vi "VisBx Anzeige_Paccar.vi"() -> ()   [LabVIEW 2020, in "Anlagenuebersicht.lvlib"]
uses:
  Seiten/Anlagenuebersicht/VisBx Anzeige/Anlagenuebersicht.lvlib
  Visualisierungs Elemente/Zahlen-Ausgabefeld.ctl
  Seiten/Anlagenuebersicht/Aktionen Ausgabefaelder einfaerben.ctl
  <vilib>/Utility/miscctls.llb/LVPointTypeDef.ctl
  Seiten/Anlagengrenzwerte/FGV Anlagengrenzwerte Aktionen.ctl
  Seiten/FT-IR/FGV FT-IR Gasliste Aktionen.ctl
  PNS/Aktionen FGV Grenzwerte.ctl
  Seiten/System Einstellungen V2/Aktioen FGV System.ctl
  Seiten/Anlagenuebersicht/VisBx Anzeige/Aktion FGV Ventile manuell schalten Crio.ctl
  Seiten/FT-IR/FGV FT-IR Diagnose Aktionen.ctl
  Messdaten/Aktionen FGV Messdaten.ctl
  Amium PNS/Aktion FGV Amium Daten.ctl
  PNS/Aktionen FGV Istwerte.ctl
  Stoerungen/Stoerungen Messgeraet/Aktionen Kommunikation Stoerung.ctl
  Funktionstasten/FGV Erweiterte Bedienung Aktion.ctl
  PNS/Aktion FGV Ventile manuell steuern.ctl
  PNS/Aktionen FGV Loopkennung.ctl
  Funktionstasten/Funktionstasten-Aktion.ctl
  <vilib>/picture/picture.llb/Draw True-Color Pixmap.vi
  Seiten/Erweiterte Konfig/Konfig CG-Check/CG-Test.vi
  Seiten/Anlagenuebersicht/VisBx Anzeige/VisBx Anzeige.lvlib
  Seiten/Anlagenuebersicht/VisBx Anzeige/TDMS laden/TDMS laden.lvlib
  Allgemein/allgemeine Sub-VIs.lvlib
  cRIO/PC/Kommunikation mit cRIO.lvlib
  Seiten/FT-IR/FT-IR.lvlib
  Stoerungen/Stoerungen.lvlib
  Seiten/Anlagengrenzwerte/Anlagengrenzwerte.lvlib
  Funktionstasten/Funktionstasten.lvlib
  Messdaten/Messdaten.lvlib
  PNS/PNS.lvlib
  Seiten/System Einstellungen V2/System Einstellungen V2.lvlib
  Seiten/Erweiterte Konfig/Konfig CG-Check/CG-Check Konfig.lvlib
  Amium PNS/Amium PNS.lvlib
  Amium PNS/Anlagenuebersicht_amium2.vi
  Passwortverwaltung/Passwort.lvlib
  Passwortverwaltung/FGV Passwort Aktion.ctl
panel:
  in  "21Y6":bool
  in  "Eingang 4":bool
  in  "Eingang 3":bool
  in  "Manueller Betrieb":u16(ring) caption="Manual Mode" items=["Normal Mode", "TESTMODE!!!!"]
  in  "11Y2":bool
  in  "11Y3":bool
  in  "12Y1":bool
  in  "11Y7":bool
  in  "11Y6":bool
  in  "21Y5":bool
  in  "20Y1":bool
  in  "20Y5":bool
  in  "21Y1":bool
  in  "20Y8":bool
  in  "20Y7":bool
  in  "20Y6":bool
  in  "20Y4":bool
  in  "20Y3":bool
  in  "20Y2":bool
  in  "23Y4":bool
  in  "23Y3":bool
  in  "22Y2":bool
  in  "23Y6":bool
  in  "11Y5":bool
  in  "22Y1":bool
  out "16B1":string="LS\n\n-16B1" caption="-21Y8"
  out "N2Exh 2":string="N2\nEXH"
  out "-22Y3 50l 2":string="-22Y3" caption="-21Y8"
  out "17B3 50l":string="LS\n\n-17B3" caption="-21Y8"
  out "17B2 50l":string="LS\n\n-17B2" caption="-21Y8"
  out "16B2 50l":string="LS\n\n-16B2" caption="-21Y8"
  out "16B2":string="LS\n\n-16B2" caption="-21Y8"
  out "-22Y1 50l":string="-22Y1" caption="-21Y8"
  out "-22Y1":string="-22Y1" caption="-21Y8"
  out "PR0,2":string="PR\n0,3bar"
  out "PA3":string="PA\n3"
  out "N2Exh":string="N2\nEXH"
  out "-23Y8":string="-23Y8"
  out "-21Y7":string="-21Y7"
  out "-21Y8":string="-21Y8"
  out "Umgebungstemperatur:":T1 caption="Ambient temperature:" format="%.1f"
  out "Boolesch":bool
  out "HL Ext. SP1:":T1 format="%.1f"
  in  "VFS":bool
  in  "VFS - Inaktiv":bool caption="VFS - Inactive"
  in  "VFS - FEHLER":bool caption="VFS - ERROR"
  in  "VFS - Aktiv":bool=TRUE caption="VFS - Active"
  out "kPa":T1 caption="Messgasdruck Amium"
  out "Durchflussblock":T1 caption="Durchflussblock:" format="%.1f"
  out "Druck Filterblock:":T1
  in  "CG-Test":bool caption="Dichtheitstest"
  out "Umgebungsdruck:":T1 caption="Ambient pressure:"
  out "Druck Ausgang:":T1 caption="Pressure outlet:"
  out "Durchfluss Bypass:":T1 caption="Flow Bypass:" format="%.1f"
  out "HL zu FID:":T1 format="%.1f"
  out "Filterblock PNS":T1 caption="Filterblock:" format="%.1f"
  out "Heizleitung SP2:":T1 caption="HL SP2:" format="%.1f"
  out "Heizleitung SP1:":T1 caption="HL SP1:" format="%.1f"
  out "Gaskühler 2":T1 caption="Gascooler:" format="%.1f"
  out "Gaskühler":T1 caption="Gascooler:" format="%.1f"
  out "Flow PMA:":T1 format="%.1f"
  out "Taupunkt":T1 caption="Dewpoint:" format="%.1f"
  out "Druck Kalter Block":T1 caption="Pressure Cold Block:"
  out "O2":T1 caption="O2:" format="%.2f"
  out "H2O":T1 format="%.2f"
  out "HC":T1 caption="HC:"
  in  "N2 zu PNS":bool
  out "Heizung VFE2:":T1 format="%.1f"
  out "HL Ext. SP2:":T1 format="%.1f"
  out "Schaltschrank:":T1 caption="Cabinet temperature:" format="%.1f"
  out "Druck CalGas:":T1 caption="Pressure CalGas:" format="%.1f"
  out "HL zu Filter:":T1 caption="HL to Filter:" format="%.1f"
  out "HL zu FT-IR:":T1 caption="HL to FT-IR:" format="%.1f"
  out "Filter:":T1 format="%.1f"
  out "Pumpe:":T1 caption="Pump:" format="%.1f"
  out "Betriebsstunden Pumpe:":T1 caption="Operating hours (measure):" format="%.1f"
  out "Betriebsstunden Anlage:":T1 caption="Operating hours (unit / FT-IR):" format="%.1f"
  out "Temp. Messzelle:":T1 caption="Temp. Gascell:" format="%.1f"
  out "Eingangsdruck FT-IR:":T1 caption="Pressure FT-IR:" format="%.3f"
  out "Durchfluss FT-IR:":T1 caption="Flow FT-IR:" format="%.1f"
  out "Aktive Störungen":string[](array[string]) caption="Errors"
  in  "Fehler":string="Die Umgebungsvariable besitzt\nnicht den selben Datentyp wie\ndie TDMS-Datei."
  out "Bild":picture
  # "Process Chart"
  # "-23Y6"
  # "-35B5"
  # "-23Y3"
  # "SPAN 1"
  # "PS"
  # "-22Y2"
  # "0-10"
  # "-20Y2"
  # "bar"
  # "-23Y4"
  # "SPAN 2"
  # "N2.....Nitrogen gaseous\nCA.....Compressed air\nCG.....Cal. Gas\nAA.....Ambient air\nPA.....Purge air FT-IR\nZG.....ZeroGas\n\nPR....Pressure regulator\nPS....Pressure switch\nFS....Flow controller\nLS....Levelsensor\nFM...Flow Sensor"
  # "PR12"
  # "-17S5"
  # "-35B1"
  # "-20Y3"
  # "SPAN 3"
  # "FM"
  # "-43Y1"
  # "-20Y4"
  # "S"
  # "SPAN 4"
  # "-21Y5"
  # "FTIR"
  # "-20Y5"
  # "SPAN 5"
  # "-20Y6"
  # "SPAN 6"
  # "-20Y7"
  # "SPAN 7"
  # "Reservoir 5l"
  # "-20Y8"
  # "SPAN 8"
  # "-35B2"
  # "-21Y1"
  # "ZeroGas"
  # "-11Y7"
  # "-11Y3"
  # "SP1"
  # "-11Y5"
  # "-11Y6"
  # "SP2"
  # "-11Y2"
  # "-12Y1"
  # "Exhaust"
  # "7A1"
  # "P out"
  # "CA to PNS"
  # "-17B8"
  # "CA in"
  # "min 4bar"
  # "-20Y1"
  # "PR01"
  # "-17S1"
  # "Purge in"
  # "-21Y6"
  # "-20Y8"
  # "°C"
  # "°C"
  # "-44Y1"
  # "-21Y8"
  # "-23Y8"
  # "-21Y7"
  # "°C"
  # "mbar"
  # "-10M2"
  # "-20Y2"
  # "°C"
  # "-20Y4"
  # "-20Y6"
  # "-7M8"
  # "-35B10"
  # "-35B6"
  # "OP"
  # "1"
  # "PS"
  # "1bar"
  # "PR"
  # "2bar"
  # "CG"
  # "PNS"
  # "SPAN 1"
  # "-23Y1"
  # "SPAN 2"
  # "PS"
  # "-23Y2"
  # "SPAN 3"
  # "0-10"
  # "bar"
  # "-23Y3"
  # "-35B5"
  # "N2.....Nitrogen gaseous\nCA.....Compressed air\nCG.....Cal. Gas\nAA.....Ambient air\nPA.....Purge air FT-IR\n\nPR....Pressure regulator\nPS....Pressure switch\nFS....Flow controller\nLS....Levelsensor\nFM...Flow Sensor"
  # "-23Y4"
  # "-21Y5"
  # "-11Y7"
  # "-11Y3"
  # "SP1"
  # "-11Y5"
  # "-11Y6"
  # "SP2"
  # "-11Y2"
  # "-12Y1"
  # "-11Y8"
  # "EPR"
  # "5bar"
  # "CA"
  # "PNS"
  # "CG"
  # "PNS"
  # "N2"
  # "4-5"
  # "CG"
  # "PNS"
  # "N2"
  # "1"
  # "PR"
  # "2bar"
  # "PS"
  # "1bar"
  # "FS"
  # "3l"
  # "PR51"
  # "N2"
  # "1-2"
  # "LS"
  # "°C"
  # "CA"
  # "6"
  # "EPR"
  # "5bar"
  # "CA"
  # "PNS"
  # "ZG"
  # "2"
  # "CG"
  # "PNS"
  # "ZG"
  # "1"
  # "PR"
  # "2bar"
  # "PS"
  # "1bar"
  # "FS"
  # "3l"
  # "PR51"
  # "N2"
  # "1-2"
  # "OP"
  # "1"
  # "CA"
  # "1-2"
  # "CA"
  # "1"
  # "ZG"
  # "2"
  # "CA"
  # "2"
  # "ZG"
  # "1"
  # "FID"
  # "EXH"
  # "°C"
  # "°C"
  # "mbar"
  # "mbar"
  # "l/min"
  # "°C"
  # "FID"
  # "EXH"
  # "M2"
  # "PR02"
  # "PR"
  # "4bar"
  # "CA"
  # "FID"
  # "M6"
  # "PR06"
  # "M7"
  # "PR07"
  # "H2"
  # "FID"
  # "PR"
  # "1,2bar"
  # "SA"
  # "FID"
  # "PR"
  # "1,2bar"
  # "-27Y4"
  # "-27Y3"
  # "PR09"
  # "-35B8"
  # "CG"
  # "O2"
  # "PS"
  # "3,5bar"
  # "FR"
  # "1,5l"
  # "FID"
  # "FID"
  # "EXH"
  # "4 bar"
  # "CA"
  # "1,2bar"
  # "H2"
  # "1,2bar"
  # "SA"
  # "SPAN 2"
  # "SPAN 3"
  # "°C"
  # "°C"
  # "°C"
  # "°C"
  # "°C"
  # "l/min"
  # "°C"
  # "mbar"
  # "H"
  # "S"
  # "P"
  # "abs"
  # "PMD"
  # "%"
  # "-35B9"
  # "FM"
  # "S"
  # "-27Y2"
  # "CG O2"
  # "CG"
  # "O2"
  # "%"
  # "ppm"
  # "°C"
  # "°C"
  # "°C"
  # "bar"
  # "°C"
  # "°C"
  # "°C"
  # "°C"
  # "h"
  # "h"
  # "°C"
  # "atm"
  # "l/min"
  # "PR"
  # "5bar"
  # "PS"
  # "4bar"
  # "P"
  # "abs"
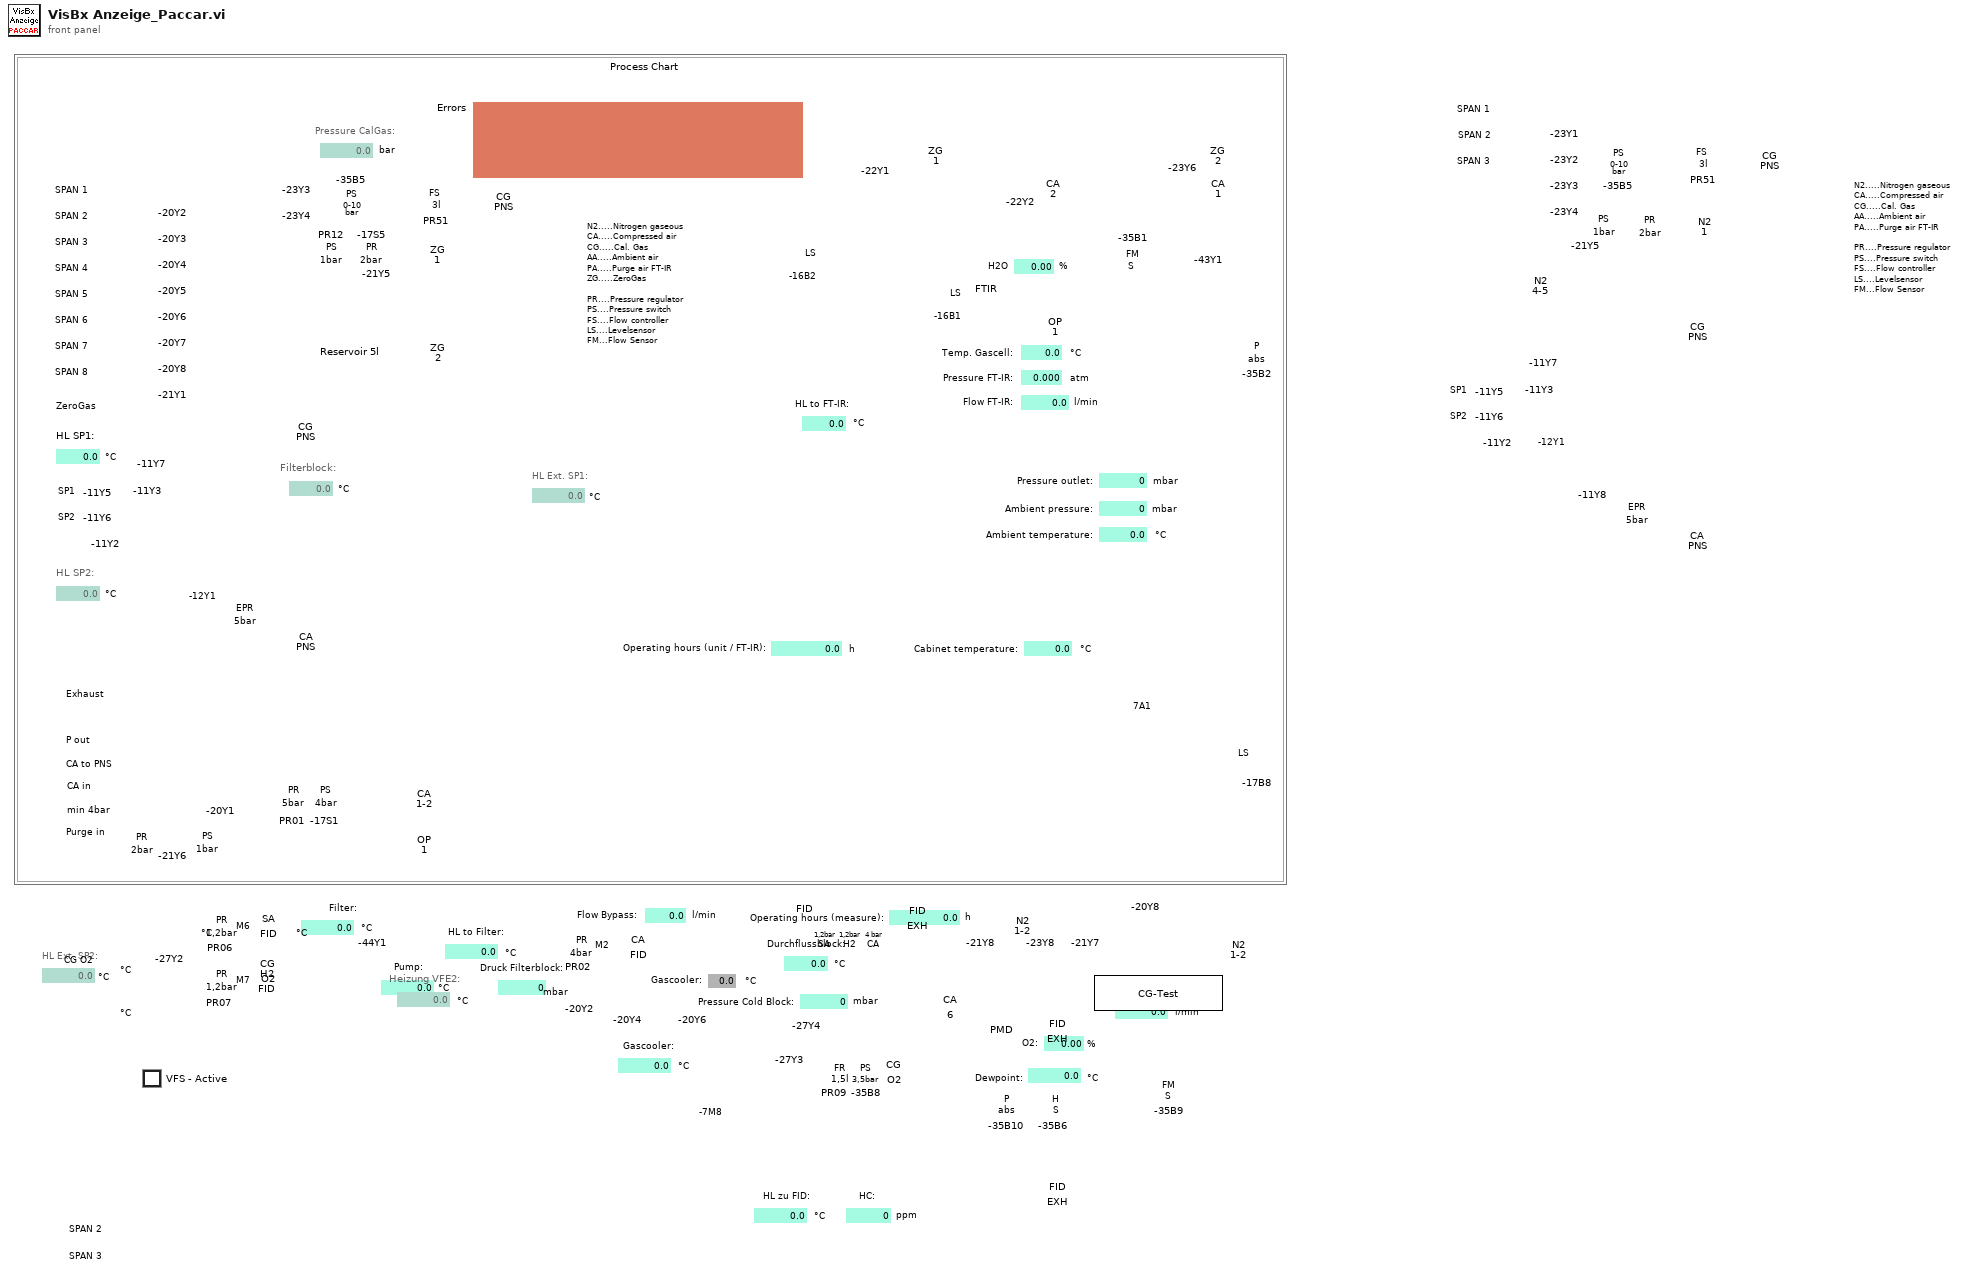
[diagram p1: front panel]
types:
  T1 = typedef "Zahlen-Ausgabefeld.ctl" = sgl
  T2 = typedef "Anlagenuebersicht.lvlib/Aktion FGV Ventile manuell schalten Crio.ctl" = enum16{"lesen", "Ventile schalten", "Testbetrieb aktiv", "Testbetrieb inaktiv", "Anzeige Ventilstellung"}
  T3 = typedef "System Einstellungen V2.lvlib/Aktioen FGV System.ctl" = enum16{"lesen", "laden", "speichern", "Optionen schreiben", "Zeitstempel", "Reset BMP", "Reset SQP", "Wartung", "Werkseinstellung"}
  T4 = typedef "PNS.lvlib/Aktionen FGV Grenzwerte.ctl" = enum16{"lesen", "Grenzw. schreiben", "Anweisungscode", "IP-Adresse", "laden", "speichern", "Anweisungscode vorgeben"}
  T5 = typedef "FT-IR.lvlib/FGV FT-IR Gasliste Aktionen.ctl" = enum16{"lesen", "Gasliste FT-IR", "Gasliste ausgelesen", "laden", "speichern", "löschen"}
  T6 = typedef "Anlagengrenzwerte.lvlib/FGV Anlagengrenzwerte Aktionen.ctl" = enum16{"Lesen", "Grenzwerte schreiben"}
  T7 = typedef "LVPointTypeDef.ctl" = cluster{"Horizontal":i16, "Vertical":i16}
  T8 = typedef "Anlagenuebersicht.lvlib/Aktionen Ausgabefaelder einfaerben.ctl" = enum16{"lesen", "prüfen", "initialisieren"}
  T9 = typedef "Funktionstasten.lvlib/FGV Erweiterte Bedienung Aktion.ctl" = enum16{"Lesen", "Initialisieren", "N2 zu PNS", "Chart wechsel"}
  T10 = typedef "Passwort.lvlib/FGV Passwort Aktion.ctl" = enum16{"prüfen", "setzen", "Initialisieren", "PW speichern", "lesen", "PW Änderung"}
  T11 = enum8{"Enabled", "Disabled", "Disabled and Grayed Out"}
  T12 = typedef "Steuerung PNS.lvclass/Anlegengrenzwerte PNS.ctl" = cluster{"Filter:":T13, "Ventilplatte:":T13, "Heizleitung 1:":T13, "Heizleitung 2:":T13, "Heizleitung 3:":T13, "Heizleitung 4:":T13, "Heizleitung 5:":T13, "Heizleitung 6:":T13}
  T13 = typedef "Steuerung PNS.lvclass/Anlagengrenzwerte Parameteranzeige.ctl" = cluster{"Sollwert":T14, "Warn-Min":T14, "Warn-Max":T14, "Abschalt-Min":T14, "Abschalt-Max":T14, "Regler":u16, "AnlagenParameter":string}
  T14 = typedef "Zahlen-Eingabefeld.ctl" = sgl
  T15 = typedef "Anlagengrenzwerte.lvlib/Anlagen-Grenzwerte Anzeige.ctl" = cluster{"Eingangsdruck FT-IR:":T16, "Durchfluss FT-IR:":T16, "Durchfluss CalGas:":T16, "Druck Ausgang:":T16, "Druck Kalter Block:":T16, "Heizleitungen intern:":T16, "Heizleitung zu FT-IR:":T16, "Heizung Filterblock:":T16, "Heizung Pumpe:":T16, "Heizleitung Extern SP1:":T16, "Heizleitung Extern SP2:":T16, "FT-IR Heizung Messzelle:":T16, "Schaltschranktemperatur:":T16, "Gaskühler:":T16}
  T16 = typedef "Anlagengrenzwerte.lvlib/Anlagen-Parameter Anzeige.ctl" = cluster{"Sollwert":sgl, "Warn-Min":sgl, "Warn-Max":sgl, "Abschalt-Min":sgl, "Abschalt-Max":sgl, "Regler":u16}
  T17 = typedef "System Einstellungen V2.lvlib/Optionen.ctl" = cluster{"Störmeldep.":bool, "Betriebszustände":bool, "AK in ppm":bool, "log Cal-Gas":bool, "log 0-Gas":bool, "Durchflusssensor 0-5V":bool, "PNS?":bool, "Mit N2 spülen":bool, "TRE08":bool, "Amium 10-Fach":bool, "Verticale Scrollbar aktiv":bool, "Loggingtakt":bool, "AK Rezeptwechsel gleich wie MKS":bool, "NG ECO":bool}
  T18 = typedef "VisParam-Typdef.lvlib/VisSchritt.ctl" = cluster{"Schritt-Typ":T19, "Schritt-Daten":variant}
  T19 = typedef "VisParam-Typdef.lvlib/VisSchritt-Typ.ctl" = enum16{"leer", "Punkt", "Linie", "Linienzug", "Fixtext", "Textrechteck", "Ziffernanzeige", "Rechteck", "Rechteck rund", "Ellipse", "Bogen", "Kreis", "Pixmap"}
  T20 = typedef "Anlagenuebersicht.lvlib/VisBx Anzeige.lvlib/TDMS laden.lvlib/TDMS-Eigenschaften.ctl" = cluster{"Größe":T21, "URL":string, "Raster":i16, "Hintergrund":u32}
  T21 = typedef "LVBoundsTypeDef.ctl" = cluster{"Width":u32, "Height":u32}
  T22 = typedef "String - Ausgabefeld.ctl" = string
  T23 = typedef "PNS.lvlib/Aktionen FGV Istwerte.ctl" = enum16{"lesen", "initialisieren", "schreiben", "Störungen"}
  T24 = typedef "Amium PNS.lvlib/Aktion FGV Amium Daten.ctl" = enum16{"lesen", "Komm Daten", "Daten", "Error", "Regler", "Grenzwerte", "laden", "speichern"}
  T25 = typedef "Messdaten.lvlib/Aktionen FGV Messdaten.ctl" = enum16{"lesen", "schreiben", "löschen", "Mittelwerte", "Komponente"}
  T26 = typedef "FT-IR.lvlib/FGV FT-IR Diagnose Aktionen.ctl" = enum16{"Lesen", "Diagnose Schreiben", "Min Schreiben", "Max Schreiben"}
  T27 = typedef "Stoerungen.lvlib/Aktionen Kommunikation Stoerung.ctl" = enum16{"lesen", "init", "FT-IR Komm", "FT-IR Betriebsart", "FT-IR Hintergrund", "cRIO Komm", "PNS Komm", "Dichtheitstest", "Life Bit", "FTIR Komm AK", "PMA Komm", "FID Komm", "PMA Cal", "FID Ch4 Cal", "FID THC Cal", "Cal Timeout", "VFS 1 Komm", "VFS 2 Komm", "VFS 3 Komm", "VFS 4 Komm", "TRE 08 Komm", "CG-Test vorzeitig", "CG-Test Span 1", "CG-Test Span 2", "CG-Test Span 3", "CG-Test Messgas", "CG-Test löschen", "Test", "Amium AK", "AK Recept konfig", "AK Name konfig", "AK EKFG konfig"}
  T28 = typedef "Funktionstasten.lvlib/Funktionstasten-Aktion.ctl" = enum16{"Initialisieren", "Zustand setzen", "Taste gedrückt", "Fehler speichern", "Lesen", "Manuell", "Remote", "Bitparallel", "Samplepoint", "Zeit Prüfen", "reset Umschalten"}
  T29 = typedef "PNS.lvlib/Aktionen FGV Loopkennung.ctl" = enum16{"lesen", "schreiben"}
  T30 = typedef "PNS.lvlib/Aktion FGV Ventile manuell steuern.ctl" = enum16{"lesen", "Ventile schalten"}
  T31 = typedef "Stoerungen.lvlib/Stoerungen Messgeraete.ctl" = cluster{"FT-IR Komm":bool, "FT-IR Betriebsart":bool, "FT-IR Hintergrundscan":bool, "Dichtheitstest":bool, "cRIO Komm":bool, "PNS Komm":bool, "Life Bit":bool, "FT-IR AK Komm":bool, "PMA Komm":bool, "FID Komm":bool, "PMA Cal":bool, "FID CH4 Cal":bool, "FID THC Cal":bool, "Cal Timeout":bool, "VFS 1 Komm":bool, "VFS 2 Komm":bool, "VFS 3 Komm":bool, "VFS 4 Komm":bool, "TRE 08 Komm":bool, "CG-Test":bool, "CG-Test 1":bool, "CG-Test 2":bool, "CG-Test 3":bool, "Messgas - Eingang":bool, "Amium AK Komm":bool, "AK Rezept nicht konfiguriert ":bool, "AK Name nicht konfiguriert":bool, "AK EKFG nicht konfiguriert":bool}
  T32 = typedef "Steuerung PNS.lvclass/Regler.ctl" = cluster{"Istwert":i16, "Sollwert":i16, "Alarm MIN":i16, "Alarm MAX":i16, "Regler sperren":i16, "Analog Ausgang":i16}[]
  T33 = typedef "Verwaltung - cRIO.lvlib/Analog Eingaenge.ctl" = cluster{"AI0: Durchfluss FT-IR":sgl, "AI1: Druck Ausgang":sgl, "AI2: Umgebungsdruck":sgl, "AI3: Druck FT-IR":sgl, "AI4: Druck CalGas":sgl, "AI5: Reserve":sgl, "AI6: Reserve":sgl, "AI7: Reserve":sgl, "Rohwert Durchfluss FT-IR":sgl, "Rohwert Druck Ausgang":sgl, "Rohwert Umgebungsdruck":sgl, "Rohwert Druck FT-IR":sgl, "Rohwert Druck CalGas":sgl, "Rohwert AI5":sgl, "Rohwert AI6":sgl, "Rohwert AI7":sgl, "Rohwert Diffdruck mbar FTIR":sgl}
  T34 = typedef "Verwaltung - cRIO.lvlib/TC Eingaenge.ctl" = cluster{"TC0: Reserve":sgl, "TC1: HL zu FT-IR":sgl, "TC2: HL Extern SP1":sgl, "TC3: HL Extern SP2":sgl, "TC4: Reserve":sgl, "TC5: Reserve":sgl, "TC6: Reserve":sgl, "TC7: Reserve":sgl, "TC8: FT-IR":sgl, "TC9: Reserve":sgl, "TC10: Schaltschrank":sgl, "TC11: Umgebung":sgl}
  T35 = typedef "Amium PNS.lvlib/Daten Cluster.ctl" = cluster{"Amium Zustände":T36, "Samplepoint am PNS":i16, "Gerätekennung":string, "aktiver Samplepoint":i16[], "Messgasdruck":sgl}
  T36 = typedef "Amium PNS.lvlib/Amium Zustand.ctl" = u16
  T37 = cluster{"Istwert":i16, "Sollwert":i16, "Alarm MIN":i16, "Alarm MAX":i16, "Regler sperren":i16, "Analog Ausgang":i16}
  T38 = typedef "Verwaltung - cRIO.lvlib/Digital Ausgaenge 0-31.ctl" = cluster{"O0: Druckluft Versorgung":bool, "O1: CG 1 (FB Eingang 1)":bool, "O2: CG 2 (Kühlung FT-IR EIN)":bool, "O3: CG 3 (FB Bypass)":bool, "O4: CG 4 (FB CalGas)":bool, "O5: CG 5 (FB spülen/UL)":bool, "O6: CG 6 (FB zum FT-IR)":bool, "O7: CG 7 (FB zum FID)":bool, "O8: CG 8 (FB Reserve)":bool, "O9: (FB Reserve)":bool, "O10: (FB Umgebungsluft FID)":bool, "O11: (FB zum Gaskühler)":bool, "O12: FB Stickstoff zu FT-IR":bool, "O13: Optikbox FT-IR spülen":bool, "O14: (Purifier deaktivieren)":bool, "O15: (Umschaltung Purifier/Stickstoff)":bool, "O16: N2 Einblasung":bool, "O17: LSP LN2 Nachfüllung":bool, "O18: (Reserve)":bool, "O19: (Pumpe Eingang1)":bool, "O20: (Pumpe Eingang2)":bool, "O21: (Pumpe Spülen1)":bool, "O22: (Pumpe Spülen2)":bool, "O23: (Reserve)":bool, "O24: CalGas 1":bool, "O25: CalGas 2":bool, "O26: CG 3-8 (CalGas 3)":bool, "O27: Stickstoff aufschalten":bool, "O28: CG zu PNS":bool, "O29: FTIR Standby Spülung":bool, "O30: CG zu Entnahme(T90)":bool, "O31: (Purifier regenerieren)":bool}
  T39 = typedef "Funktionstasten.lvlib/Zustaende.ctl" = enum16{"Standby", "Pause", "Eco", "Messen", "Kalibrieren", "Spülen Filter", "Spülen Leitung", "Umgebungsluft", "0-Gas", "Cal-Gas", "CG zu PNS", "-------------", "Init 1", "Init 2", "Init 3", "Init 4", "Messen vorbereiten", "Messen durchführen", "Exit"}
  T40 = typedef "PNS.lvlib/PNS Geraetekennung.ctl" = cluster{"Loops":string[], "Gerätetype":string, "Loopkennung":u16[], "Seriennummer":string, "Geraetekennung":u16, "SoftWare Version":string, "LP Kennung":u16}
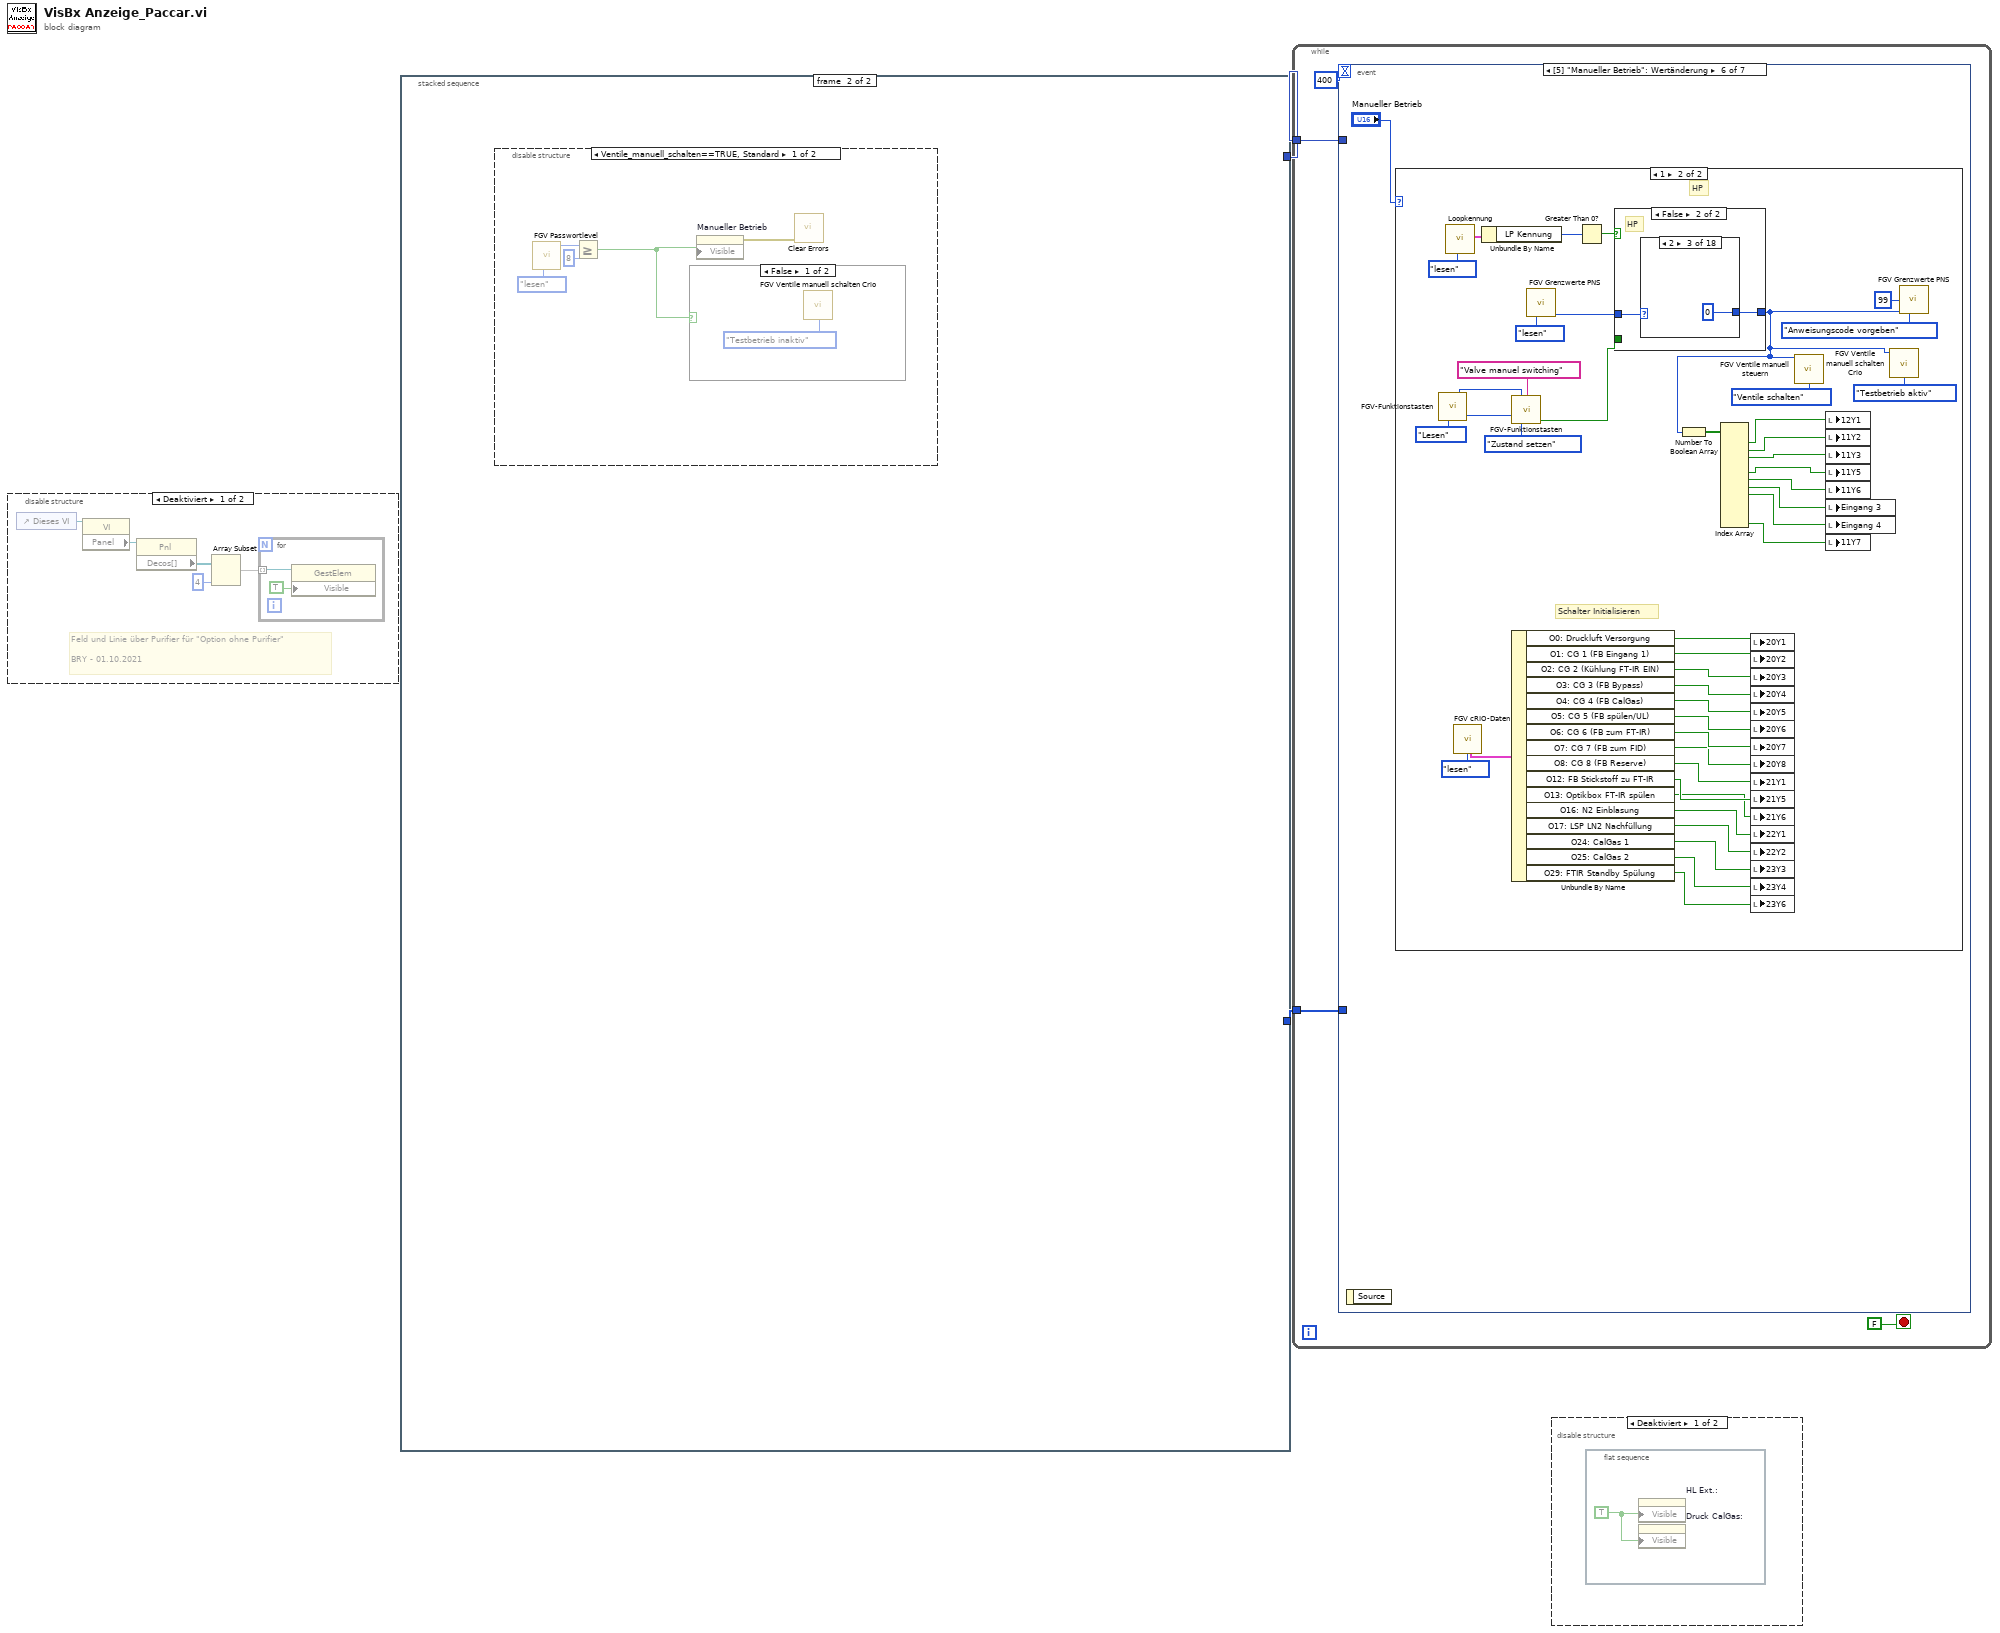
[diagram p0: block diagram]
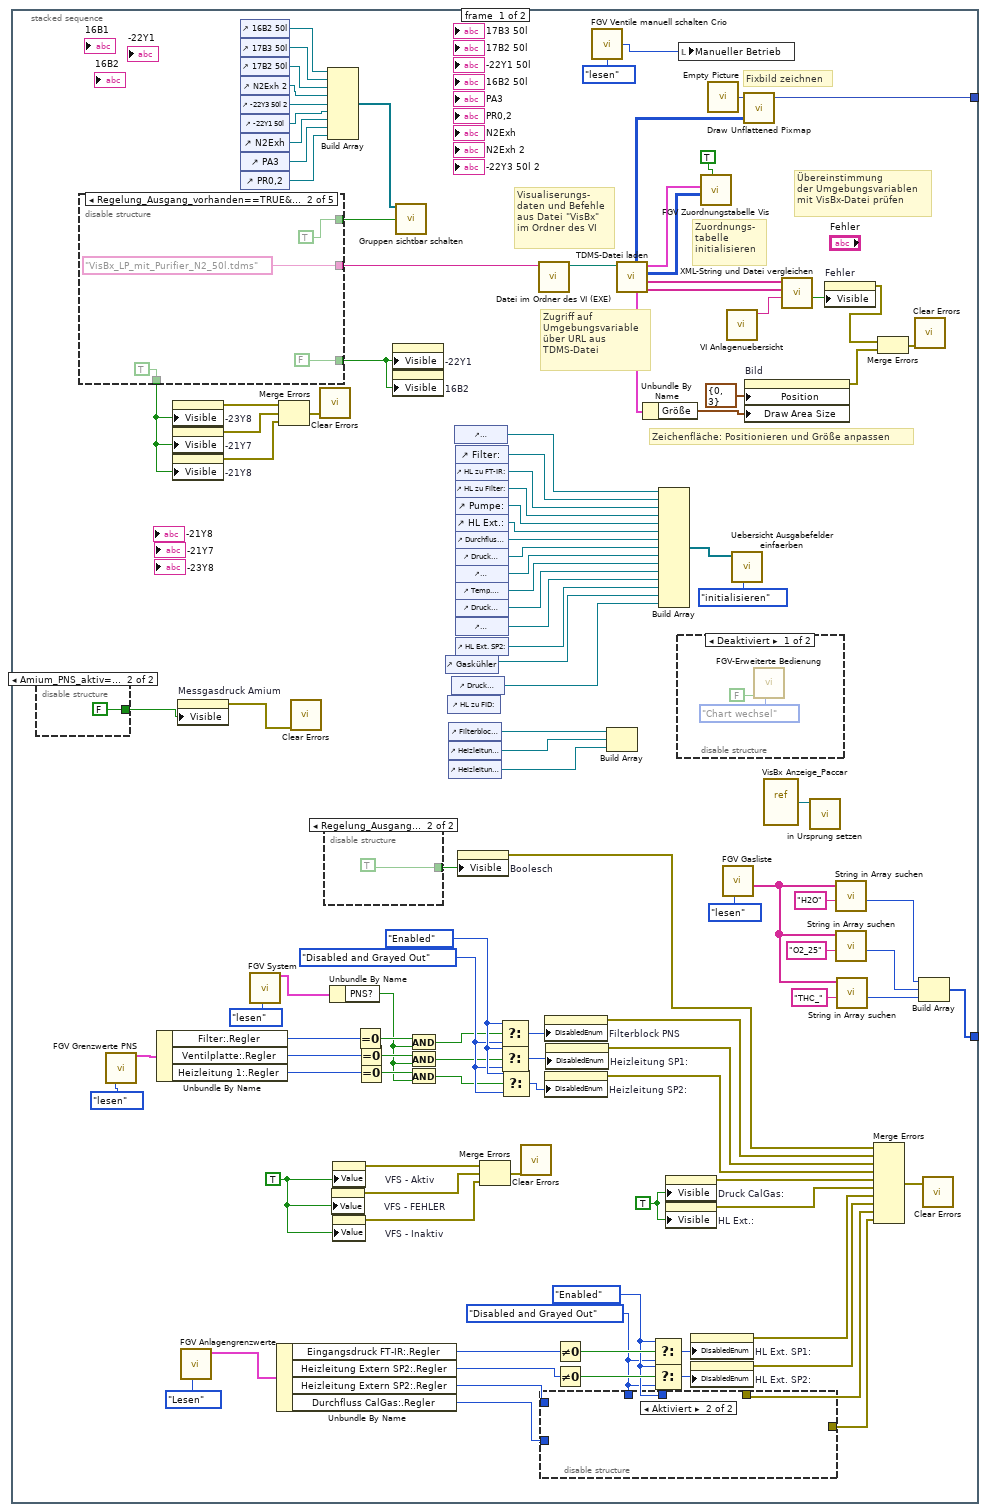
[diagram p2: hidden frame]
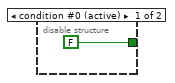
[diagram p3: hidden frame]
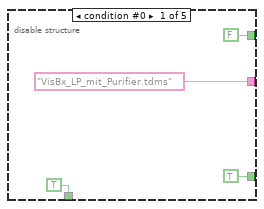
[diagram p4: hidden frame]
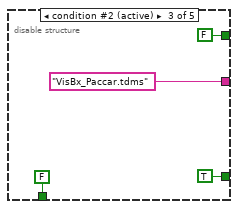
[diagram p5: hidden frame]
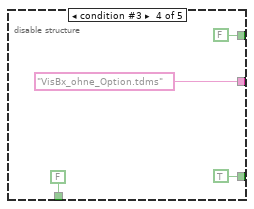
[diagram p6: hidden frame]
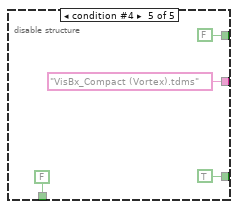
[diagram p7: hidden frame]
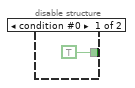
[diagram p8: hidden frame]
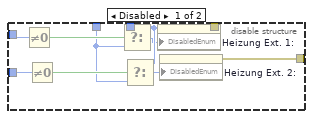
[diagram p9: hidden frame]
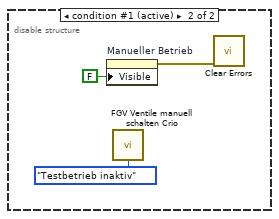
[diagram p12: hidden frame]
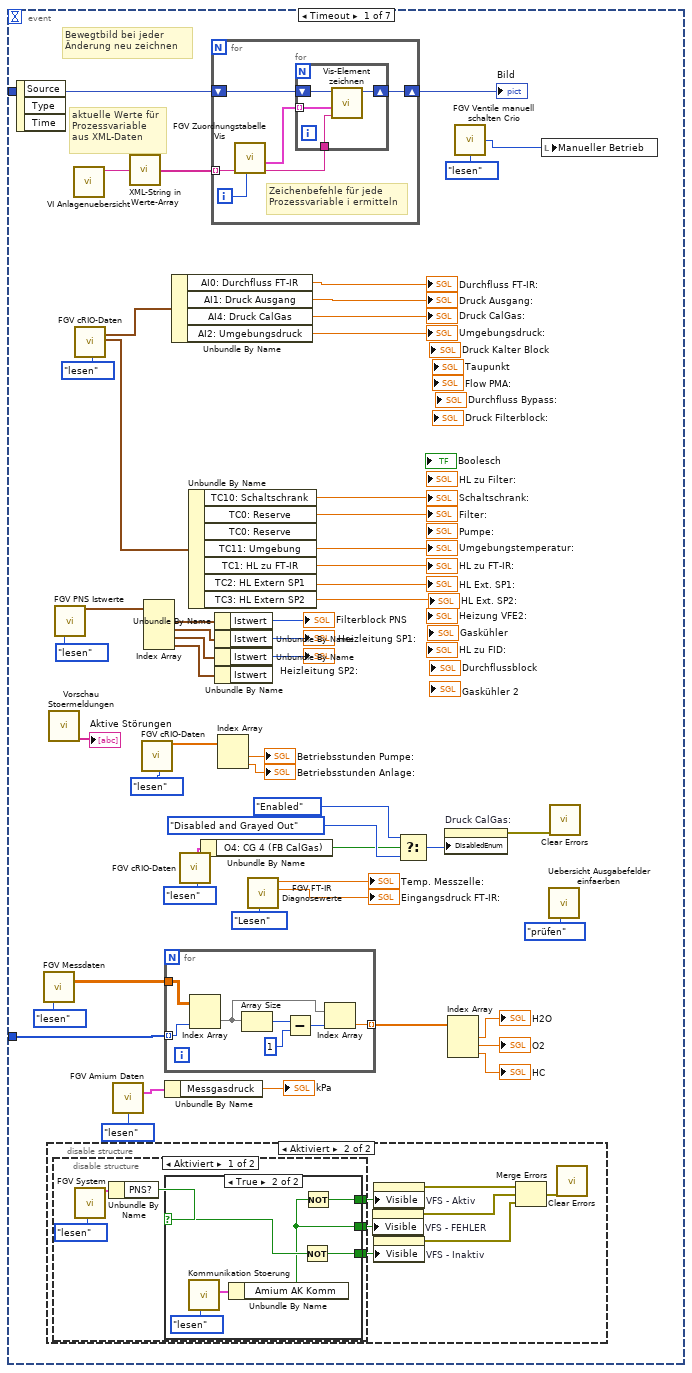
[diagram p15: hidden frame]
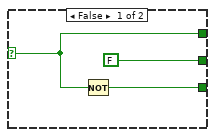
[diagram p17: hidden frame]
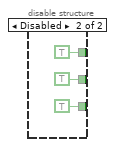
[diagram p18: hidden frame]
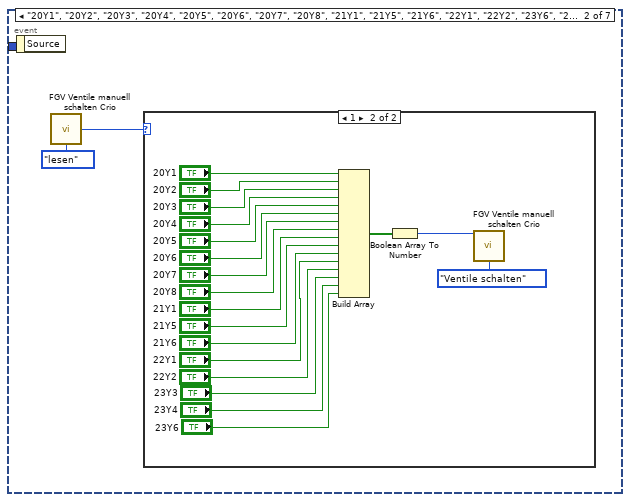
[diagram p19: hidden frame]
diagram:
  n1 = disable-structure shown="Deaktiviert" {
    frame Disabled {
      # "Feld und Linie über Purifier für \"Option ohne Purifier\"\n\nBRY - 01.10.2021"
      n2 = control-ref of="Dieses VI"() -> (w7:refnum<vi>)
      n3 = property class="VI"(reference=w7) -> ("Panel"=w6:refnum<vi>)  [unwired: 1 in, 2 out]
      n4 = property class="Pnl"(reference=w6) -> ("Decos[]"=w5:refnum<vi>[])  [unwired: 1 in, 2 out]
      n5 = Array Subset(array=w5, length=4 ("Länge")) -> (w3:refnum<vi>[])  [unwired: 1 in]
      n6 = for {
        tunnel: w3 -> [w9] mode=indexing
        n7 = property class="GestElem"(reference=w9, "Visible"=TRUE ("Sichtbar")) -> ()  [unwired: 1 in, 2 out]
      }
    }
    frame Enabled {
    }
  }
  n8 = stacked-sequence {
    tunnel: [w101 _] -> w2
    tunnel: [w68 _] -> w1
    frame #0 {
      w34 = TRUE ("Sichtbar")
      w53 = T11."Enabled" ("t")
      w52 = T11."Disabled and Grayed Out" ("Deaktiviert")
      w82 = T11."Enabled" ("t")
      w81 = T11."Disabled and Grayed Out" ("Deaktiviert")
      w94 = TRUE ("Sichtbar")
      # "Übereinstimmung\nder Umgebungsvariablen\nmit VisBx-Datei prüfen"
      # "Zugriff auf\nUmgebungsvariable\nüber URL aus\nTDMS-Datei"
      # "Visualiserungs-\ndaten und Befehle\naus Datei \"VisBx\"\nim Ordner des VI"
      # "Zuordnungs-\ntabelle\ninitialisieren"
      # "Zeichenfläche: Positionieren und Größe anpassen"
      # "Fixbild zeichnen"
      n9 = disable-structure shown="Amium_PNS_aktiv==FALSE, Standard" {
        disable-tunnel: [TRUE FALSE] -> w33
        frame condition #0 {
        }
        frame condition #1 (active) {
        }
      }
      n10 = disable-structure shown="Regelung_Ausgang_vorhanden==TRUE&&LN2_Befuellung==TRUE&&Purifier==TRUE&&50l_N2_Tank==TRUE" {
        disable-tunnel: ["VisBx_LP_mit_Purifier.tdms" ("Dateiname") "VisBx_LP_mit_Purifier_N2_50l.tdms" ("Dateiname") "VisBx_Paccar.tdms" ("Dateiname") "VisBx_ohne_Option.tdms" ("Dateiname") "VisBx_Compact (Vortex).tdms" ("Dateiname")] -> w31
        disable-tunnel: [TRUE ("Sichtbar") TRUE ("Sichtbar") FALSE ("Sichtbar") FALSE ("Sichtbar") FALSE ("Sichtbar")] -> w28
        disable-tunnel: [TRUE ("Sichtbar") FALSE ("Sichtbar") TRUE ("Sichtbar") TRUE ("Sichtbar") TRUE ("Sichtbar")] -> w23
        disable-tunnel: [FALSE ("Sichtbar") TRUE ("Sichtbar") FALSE ("Sichtbar") FALSE ("Sichtbar") FALSE ("Sichtbar")] -> w12
        frame condition #0 {
        }
        frame condition #1 {
        }
        frame condition #2 (active) {
        }
        frame condition #3 {
        }
        frame condition #4 {
        }
      }
      n11 = call "FGV Grenzwerte PNS.vi"("Aktionen FGV Grenzwerte"=Aktionen_FGV_Grenzwerte."lesen") -> ("Grenzwerte PNS 2"=w64:T12)  [unwired: 12 in, 2 out]
      n12 = Unbundle By Name(w64) -> ("Filter:.Regler"=w62:u16, "Ventilplatte:.Regler"=w61:u16, "Heizleitung 1:.Regler"=w60:u16)
      n13 = property on="-23Y8" class="Str"("Visible"=w28) -> (error out=w27:errorcluster)  [unwired: 2 in, 1 out]
      n14 = property on="-21Y7" class="Str"("Visible"=w28) -> (error out=w26:errorcluster)  [unwired: 2 in, 1 out]
      n15 = property on="-21Y8" class="Str"("Visible"=w28) -> (error out=w25:errorcluster)  [unwired: 2 in, 1 out]
      n16 = property on="Messgasdruck Amium" class="DigWert (strikt)"("Visible"=w33) -> (error out=w32:errorcluster)  [unwired: 2 in, 1 out]
      n17 = call "FGV Anlagengrenzwerte.vi"("Aktion"=FGV_Anlagengrenzwerte_Aktionen."Lesen") -> ("Anlagen-Grenzwerte Anzeige"=w91:T15)  [unwired: 1 in, 9 out]
      n18 = control-ref of="16B2 50l"() -> (w22:refnum<vi>)
      n19 = control-ref of="17B3 50l"() -> (w21:refnum<vi>)
      n20 = control-ref of="17B2 50l"() -> (w20:refnum<vi>)
      n21 = control-ref of="N2Exh 2"() -> (w19:refnum<vi>)
      n22 = control-ref of="-22Y3 50l 2"() -> (w18:refnum<vi>)
      n23 = control-ref of="-22Y1 50l"() -> (w17:refnum<vi>)
      n24 = control-ref of="N2Exh"() -> (w16:refnum<vi>)
      n25 = control-ref of="PA3"() -> (w15:refnum<vi>)
      n26 = control-ref of="PR0,2"() -> (w14:refnum<vi>)
      n27 = call "FGV System.vi"("Aktionen"=Aktioen_FGV_System."lesen") -> ("Optionen"=w55:T17)  [unwired: 12 in, 6 out]
      n28 = Unbundle By Name(w91) -> ("Eingangsdruck FT-IR:.Regler"=w89:u16, "Heizleitung Extern SP2:.Regler"=w85:u16, "Heizleitung Extern SP2:.Regler"=w83:u16, "Durchfluss CalGas:.Regler"=w80:u16)
      n29 = Merge Errors(w27, w26, w25) -> (w24:errorcluster)
      n30 = call <vilib>:"Clear Errors.vi"("error in (no error)"=w32) -> ()  [unwired: 5 in, 2 out]
      n31 = call <vilib>:"Clear Errors.vi"("error in (no error)"=w24) -> ()  [unwired: 5 in, 2 out]
      n32 = disable-structure shown="Regelung_Ausgang_vorhanden==FALSE" {
        disable-tunnel: [FALSE ("Sichtbar") TRUE ("Sichtbar")] -> w30
        frame condition #0 (active) {
        }
        frame condition #1 {
        }
      }
      n33 = Build Array(w22, w21, w20, w19, w18, w17, w16, w15, w14) -> (w13:refnum<vi>[])
      n34 = Unbundle By Name(w55) -> ("PNS?"=w54:bool)
      n35 = property on="VFS - FEHLER" class="Bool. (strikt)"("Value"=w34) -> (error out=w36:errorcluster)  [unwired: 2 in, 1 out]
      n36 = property on="VFS - Aktiv" class="Bool. (strikt)"("Value"=w34) -> (error out=w37:errorcluster)  [unwired: 2 in, 1 out]
      n37 = property on="VFS - Inaktiv" class="Bool. (strikt)"("Value"=w34) -> (error out=w35:errorcluster)  [unwired: 2 in, 1 out]
      n38 = Equal To 0?(x=w62) -> (x = 0?=w59:bool)
      n39 = Equal To 0?(x=w61) -> (x = 0?=w58:bool)
      n40 = Equal To 0?(x=w60) -> (x = 0?=w57:bool)
      n41 = property on="-22Y1" class="Str"("Visible"=w23) -> ()  [unwired: 2 in, 2 out]
      n42 = property on="16B2" class="Str"("Visible"=w23) -> ()  [unwired: 2 in, 2 out]
      n43 = call "Gruppen sichtbar schalten.vi"("Element Referenzen"=w13, "Sichtbar"=w12) -> ()  [unwired: 13 in, 1 out]
      n44 = And(x=w59, y=w54) -> (x .and. y?=w51:bool)
      n45 = And(x=w58, y=w54) -> (x .and. y?=w50:bool)
      n46 = And(x=w57, y=w54) -> (x .and. y?=w49:bool)
      n47 = control-ref of="Gaskühler"() -> (w65:refnum<vi>)
      n48 = control-ref of="HL zu FID:"() -> ()  [unwired: 1 out]
      n49 = control-ref of="Filterblock PNS"() -> (w42:refnum<vi>)
      n50 = control-ref of="Heizleitung SP1:"() -> (w41:refnum<vi>)
      n51 = control-ref of="Heizleitung SP2:"() -> (w40:refnum<vi>)
      n52 = control-ref of="Druck Kalter Block"() -> (w66:refnum<vi>)
      n53 = control-ref of="Durchflussblock"() -> (w39:refnum<vi>)
      n54 = control-ref of="Filter:"() -> (w125:refnum<vi>)
      n55 = control-ref of="HL zu FT-IR:"() -> (w127:refnum<vi>)
      n56 = control-ref of="HL zu Filter:"() -> (w126:refnum<vi>)
      n57 = control-ref of="Pumpe:"() -> (w124:refnum<vi>)
      n58 = control-ref of="HL Ext.:"() -> (w123:refnum<vi>)
      n59 = control-ref of="Durchfluss FT-IR:"() -> (w122:refnum<vi>)
      n60 = control-ref of="Druck Ausgang:"() -> (w121:refnum<vi>)
      n61 = control-ref of="Eingangsdruck FT-IR:"() -> (w120:refnum<vi>)
      n62 = control-ref of="Temp. Messzelle:"() -> (w119:refnum<vi>)
      n63 = control-ref of="Druck CalGas:"() -> (w116:refnum<vi>)
      n64 = control-ref of="Schaltschrank:"() -> (w93:refnum<vi>)
      n65 = control-ref of="HL Ext. SP2:"() -> (w76:refnum<vi>)
      n66 = property on="Boolesch" class="Bool. (strikt)"("Visible"=w30) -> (error out=w29:errorcluster)  [unwired: 2 in, 1 out]
      n67 = Merge Errors(w37, w36, w35) -> (w38:errorcluster)
      n68 = Select(t=w53, s=w51, f=w52) -> (s? t:f=w48:T11)
      n69 = Select(t=w53, s=w50, f=w52) -> (s? t:f=w47:T11)
      n70 = Select(t=w53, s=w49, f=w52) -> (s? t:f=w46:T11)
      n71 = call <vilib>:"Clear Errors.vi"("error in (no error)"=w38) -> ()  [unwired: 5 in, 2 out]
      n72 = call "Datei im Ordner des VI (EXE).vi"("Dateiname"=w31) -> ("Dateipfad im Ordner des Haupt-VIs"=w114:path)  [unwired: 8 in, 2 out]
      n73 = disable-structure shown="Aktiviert" {
        disable-tunnel: w83 -> [w160 _]
        disable-tunnel: w82 -> [w158 _]
        disable-tunnel: w81 -> [w157 _]
        disable-tunnel: w80 -> [w156 _]
        disable-tunnel: [w153 _] -> w78
        disable-tunnel: [w152 _] -> w77
        frame Disabled {
          n74 = Not Equal To 0?(x=w160) -> (x != 0?=w161:bool)
          n75 = Not Equal To 0?(x=w156) -> (x != 0?=w159:bool)
          n76 = Select(t=w158, s=w161, f=w157) -> (s? t:f=w155:T11)
          n77 = Select(t=w158, s=w159, f=w157) -> (s? t:f=w154:T11)
          n78 = property on="Heizung Ext. 1:" class="DigWert (strikt)"("DisabledEnum"=w155) -> (error out=w153:errorcluster)  [unwired: 2 in, 1 out]
          n79 = property on="Heizung Ext. 2:" class="DigWert (strikt)"("DisabledEnum"=w154) -> (error out=w152:errorcluster)  [unwired: 2 in, 1 out]
        }
        frame Enabled {
        }
      }
      n80 = property on="Filterblock PNS" class="DigWert (strikt)"("DisabledEnum"=w48) -> (error out=w45:errorcluster)  [unwired: 2 in, 1 out]
      n81 = property on="Heizleitung SP2:" class="DigWert (strikt)"("DisabledEnum"=w46) -> (error out=w43:errorcluster)  [unwired: 2 in, 1 out]
      n82 = property on="Heizleitung SP1:" class="DigWert (strikt)"("DisabledEnum"=w47) -> (error out=w44:errorcluster)  [unwired: 2 in, 1 out]
      n83 = Not Equal To 0?(x=w89) -> (x != 0?=w90:bool)
      n84 = Not Equal To 0?(x=w85) -> (x != 0?=w86:bool)
      n85 = call "FGV Ventile manuell schalten Crio.vi"("Aktion"=Aktion_FGV_Ventile_manuell_schalten_Crio."lesen") -> ("Betrieb"=w10:u16)  [unwired: 11 in, 3 out]
      n86 = Build Array(w42, w41, w40) -> ()  [unwired: 1 out]
      n87 = call "TDMS-Datei laden.vi"("Dateipfad"=w114) -> ("Datentypen"=w110:string[], "Namen"=w106:string[], "Zuordnungstabelle"=w104:i16[][], "Programm"=w105:T18[], "Eigenschaften"=w107:T20, "Fixbild (Pixmap)"=w108:u32[][])  [unwired: 5 out]
      n88 = Unbundle By Name(w107) -> ("Größe"=w113:T21)
      n89 = Select(t=w82, s=w90, f=w81) -> (s? t:f=w88:T11)
      n90 = Select(t=w82, s=w86, f=w81) -> (s? t:f=w84:T11)
      n91 = Build Array(w39, w125, w127, w126, w124, w123, w122, w121, w120, w119, w116, w93, w76, w65, w66) -> (w118:refnum<vi>[])
      n92 = property on="Druck CalGas:" class="DigWert (strikt)"("Visible"=w94) -> (error out=w95:errorcluster)  [unwired: 2 in, 1 out]
      n93 = property on="HL Ext.:" class="DigWert (strikt)"("Visible"=w94) -> (error out=w96:errorcluster)  [unwired: 2 in, 1 out]
      n94 = disable-structure shown="Deaktiviert" {
        frame Disabled {
          n95 = call "FGV-Erweiterte Bedienung.vi"("Aktion"=FGV_Erweiterte_Bedienung_Aktion."Chart wechsel", "Chart wechsel"=FALSE) -> ()  [unwired: 8 in, 2 out]
        }
        frame Enabled {
        }
      }
      n96 = local write "Manueller Betrieb"(w10) -> ()
      n97 = property on="HL Ext. SP1:" class="DigWert (strikt)"("DisabledEnum"=w88) -> (error out=w87:errorcluster)  [unwired: 2 in, 1 out]
      n98 = property on="HL Ext. SP2:" class="DigWert (strikt)"("DisabledEnum"=w84) -> (error out=w79:errorcluster)  [unwired: 2 in, 1 out]
      n99 = call "FGV Zuordnungstabelle Vis.vi"("Initialisieren"=TRUE, "Zuordnungtabelle (init)"=w104, "Programm (init)"=w105) -> ()  [unwired: 3 in, 6 out]
      n100 = call "Empty Picture"() -> ("empty picture"=w109:picture)
      n101 = call "FGV Gasliste.vi"("Aktionen"=FGV_FT-IR_Gasliste_Aktionen."lesen") -> ("Aktuelle Gasliste gesamt"=w67:T22[])  [unwired: 8 in, 2 out]
      n102 = call "VI Anlagenuebersicht.vi"() -> ("XML-String"=w111:string)  [unwired: 11 in]
      n103 = call "Uebersicht Ausgabefelder einfaerben.vi"("Aktionen"=Aktionen_Ausgabefaelder_einfaerben."initialisieren", "Angehängtes Array"=w118) -> ()  [unwired: 10 in]
      n104 = call-poly <vilib>:"Draw Unflattened Pixmap.vi"("picture"=w109, "data (RGB format)"=w108) -> ("new picture"=w101:picture)  [unwired: 7 in]
      n105 = property on="Bild" class="Bild"("Position"=T7 {"Horizontal"=0, "Vertical"=3} ("Ursprung"), "Draw Area Size"=w113) -> (error out=w97:errorcluster)  [unwired: 2 in, 1 out]
      n106 = vi-ref "VisBx Anzeige_Paccar.vi"() -> (w115:refnum<vi>)
      n107 = call "XML-String und Datei vergleichen.vi"("XML-String"=w111, "Datentypen aus Datei"=w110, "Namen aus Datei"=w106) -> ("nicht gleich"=w103:bool)  [unwired: 8 out]
      n108 = call "in Ursprung setzen.vi"("VI Referenz"=w115) -> ()  [unwired: 10 in, 1 out]
      n109 = property on="Fehler" class="Str"("Visible"=w103) -> (error out=w98:errorcluster)  [unwired: 2 in, 1 out]
      n110 = call "String in Array suchen.vi"("Nach String/Zeichen suchen (-)"="H2O", "String-Array"=w67) -> ("Index"=w71:i32)  [unwired: 7 in, 2 out]
      n111 = call "String in Array suchen.vi"("Nach String/Zeichen suchen (-)"="O2_25", "String-Array"=w67) -> ("Index"=w70:i32)  [unwired: 7 in, 2 out]
      n112 = call "String in Array suchen.vi"("Nach String/Zeichen suchen (-)"="THC_", "String-Array"=w67) -> ("Index"=w69:i32)  [unwired: 7 in, 2 out]
      n113 = Merge Errors(w29, w45, w44, w43, w95, w96, w87, w79, w78, w77) -> (w100:errorcluster)
      n114 = Merge Errors(w98, w97) -> (w99:errorcluster)
      n115 = call <vilib>:"Clear Errors.vi"("error in (no error)"=w99) -> ()  [unwired: 5 in, 2 out]
      n116 = Build Array(w71, w70, w69) -> (w68:i32[])
      n117 = call <vilib>:"Clear Errors.vi"("error in (no error)"=w100) -> ()  [unwired: 5 in, 2 out]
    }
    frame #1 {
      n118 = disable-structure shown="Ventile_manuell_schalten==TRUE, Standard" {
        frame condition #0 {
          n119 = call "FGV Passwortlevel.vi"("FGV Passwort Aktion"=FGV_Passwort_Aktion."lesen") -> ("aktueller Level"=w167:i16)  [unwired: 8 in, 2 out]
          n120 = Greater Or Equal?(x=w167, y=i16 8) -> (x >= y?=w164:bool)
          n121 = case shown="False" w164 {
            frame False {
              n122 = call "FGV Ventile manuell schalten Crio.vi"("Aktion"=Aktion_FGV_Ventile_manuell_schalten_Crio."Testbetrieb inaktiv") -> ()  [unwired: 11 in, 4 out]
            }
            frame True {
            }
          }
          n123 = property on="Manueller Betrieb" class="Ring (strikt)"("Visible"=w164) -> (error out=w165:errorcluster)  [unwired: 2 in, 1 out]
          n124 = call <vilib>:"Clear Errors.vi"("error in (no error)"=w165) -> ()  [unwired: 5 in, 2 out]
        }
        frame condition #1 (active) {
          n125 = property on="Manueller Betrieb" class="Ring (strikt)"("Visible"=FALSE ("Sichtbar")) -> (error out=w171:errorcluster)  [unwired: 2 in, 1 out]
          n126 = call "FGV Ventile manuell schalten Crio.vi"("Aktion"=Aktion_FGV_Ventile_manuell_schalten_Crio."Testbetrieb inaktiv") -> ()  [unwired: 11 in, 4 out]
          n127 = call <vilib>:"Clear Errors.vi"("error in (no error)"=w171) -> ()  [unwired: 5 in, 2 out]
        }
      }
    }
  }
  n128 = while {
    tunnel: w2 -> [w176]
    tunnel: w1 -> [w173]
    stop <- FALSE stop-if-true
    n129 = event shown="[5] \"Manueller Betrieb\": Wertänderung" {
      selector: _ -> [_ _ _ _ _ _ _]
      dyn-events: _ -> [_ _ _ _ _ _ _]
      timeout: 400 -> [_ _ _ _ _ _ _]
      tunnel: w176 -> [w230 _ _ _ _ _ _]
      tunnel: w173 -> [w201 _ _ _ _ _ _]
      event Timeout {
        # "aktuelle Werte für\nProzessvariable\naus XML-Daten"
        # "Bewegtbild bei jeder\nÄnderung neu zeichnen"
        n130 = event-data() -> ()  [unwired: 1 in, 3 out]
        n131 = call "FGV Messdaten.vi"("Aktionen"=Aktionen_FGV_Messdaten."lesen") -> ("Messdaten"=w195:sgl[][])  [unwired: 6 in, 8 out]
        n132 = disable-structure shown="Aktiviert" {
          frame Disabled {
          }
          frame Enabled {
            n133 = disable-structure shown="Aktiviert" {
              disable-tunnel: [w241 TRUE] -> w237
              disable-tunnel: [w240 TRUE ("Amium AK Komm")] -> w236
              disable-tunnel: [w239 TRUE] -> w235
              frame Enabled {
                n134 = call "FGV System.vi"("Aktionen"=Aktioen_FGV_System."lesen") -> ("Optionen"=w242:T17)  [unwired: 12 in, 6 out]
                n135 = Unbundle By Name(w242) -> ("PNS?"=w238:bool)
                n136 = case shown="True" w238 {
                  selector: w238 -> [w245 w252]
                  tunnel: [w245 w247] -> w239
                  tunnel: [FALSE w248] -> w240
                  tunnel: [w244 w251] -> w241
                  frame False {
                    n137 = Not(x=w245) -> (.not. x?=w244:bool)
                  }
                  frame True {
                    n138 = call "Kommunikation Stoerung.vi"("Aktionen"=Aktionen_Kommunikation_Stoerung."lesen") -> ("Störung Messgerät"=w249:T31)  [unwired: 10 in]
                    n139 = Unbundle By Name(w249) -> ("Amium AK Komm"=w248:bool)
                    n140 = Not(x=w252) -> (.not. x?=w251:bool)
                    n141 = Not(x=w248) -> (.not. x?=w247:bool)
                  }
                }
              }
              frame Disabled {
              }
            }
            n142 = property on="VFS - FEHLER" class="Bool. (strikt)"("Visible"=w236) -> (error out=w233:errorcluster)  [unwired: 2 in, 1 out]
            n143 = property on="VFS - Aktiv" class="Bool. (strikt)"("Visible"=w235) -> (error out=w232:errorcluster)  [unwired: 2 in, 1 out]
            n144 = property on="VFS - Inaktiv" class="Bool. (strikt)"("Visible"=w237) -> (error out=w234:errorcluster)  [unwired: 2 in, 1 out]
            n145 = Merge Errors(w232, w233, w234) -> (w231:errorcluster)
            n146 = call <vilib>:"Clear Errors.vi"("error in (no error)"=w231) -> ()  [unwired: 5 in, 2 out]
          }
        }
        n147 = call "Vorschau Stoermeldungen.vi"() -> ("Vorschau Störungen"=→"Aktive Störungen":string[])  [unwired: 10 in, 1 out]
        n148 = call "FGV PNS Istwerte.vi"("Aktionen"=Aktionen_FGV_Istwerte."lesen") -> ("Regler"=w184:T32)  [unwired: 11 in, 3 out]
        n149 = call "VI Anlagenuebersicht.vi"() -> ("XML-String"=w219:string)  [unwired: 11 in]
        n150 = call "FGV cRIO-Daten.vi"("Aktion"=enum16{"lesen", "schreiben"}."lesen") -> ("Analog Input"=w223:T33, "TC Eingänge"=w204:T34)  [unwired: 9 in, 8 out]
        n151 = call "FGV Amium Daten.vi"("Aktion"=Aktion_FGV_Amium_Daten."lesen") -> ("Amium Daten"=w193:T35)  [unwired: 9 in, 5 out]
        n152 = call "XML-String in Werte-Array.vi"("XML-String"=w219) -> ("Werte"=w220:string[])
        n153 = call "FGV cRIO-Daten.vi"("Aktion"=enum16{"lesen", "schreiben"}."lesen") -> ("Betriebsstunden"=w212:sgl[])  [unwired: 9 in, 9 out]
        n154 = Index Array(array=w184) -> (element #1=w185:T37, element #2=w186:T37, element #3=w187:T37, element #4=w188:T37)  [unwired: 4 in]
        n155 = for {
          tunnel: [w259] -> w199 mode=indexing
          tunnel: w201 -> [w256] mode=indexing
          tunnel: w195 -> [w257]
          n156 = Index Array(array=w257, index (col)=w256) -> (element=w258:sgl[])  [unwired: 1 in]
          n157 = Array Size(array=w258) -> (size(s)=w262:i32)
          n158 = Subtract(x=w262, y=1) -> (x-y=w260:i32)
          n159 = Index Array(array=w258, index=w260) -> (element=w259:sgl)
        }
        n160 = Unbundle By Name(w193) -> ("Messgasdruck"=→"kPa":sgl)
        n161 = Unbundle By Name(w223) -> ("AI0: Durchfluss FT-IR"=→"Durchfluss FT-IR:":sgl, "AI1: Druck Ausgang"=→"Druck Ausgang:":sgl, "AI4: Druck CalGas"=→"Druck CalGas:":sgl, "AI2: Umgebungsdruck"=→"Umgebungsdruck:":sgl)
        n162 = call "FGV cRIO-Daten.vi"("Aktion"=enum16{"lesen", "schreiben"}."lesen") -> ("DO 0-31"=w215:T38)  [unwired: 9 in, 9 out]
        n163 = Unbundle By Name(w204) -> ("TC10: Schaltschrank"=→"Schaltschrank:":sgl, "TC0: Reserve"=→"Filter:":sgl, "TC11: Umgebung"=→"Umgebungstemperatur:":sgl, "TC1: HL zu FT-IR"=→"HL zu FT-IR:":sgl, "TC2: HL Extern SP1"=→"HL Ext. SP1:":sgl, "TC3: HL Extern SP2"=→"HL Ext. SP2:":sgl)  [unwired: 1 out]
        n164 = Unbundle By Name(w215) -> ("O4: CG 4 (FB CalGas)"=w209:bool)
        n165 = for {
          shift-right: [w268] -> w218
          shift-left: w230 -> [w265]
          tunnel: w220 -> [w264] mode=indexing
          i -> [w263]
          # "Zeichenbefehle für jede\nProzessvariable i ermitteln"
          n166 = call "FGV Zuordnungstabelle Vis.vi"("Prozessvariable Nr. N"=w263, "Wert (N)"=w264) -> ("Wert für zeichnen"=w266:string, "Zeichenbefehle"=w267:T18[])  [unwired: 4 in, 4 out]
          n167 = for {
            tunnel: w266 -> [w269]
            tunnel: w267 -> [w270] mode=indexing
            shift-right: [w272] -> w268
            shift-left: w265 -> [w271]
            n168 = call "Vis-Element zeichnen.vi"("Wert-String"=w269, "Schritt"=w270, "Bild alt"=w271) -> ("Bild neu"=w272:picture)  [unwired: 4 in, 4 out]
          }
        }
        "Bild" <- w218
        n169 = Unbundle By Name(w185) -> ("Istwert"=→"Filterblock PNS":i16)
        n170 = Unbundle By Name(w186) -> ("Istwert"=→"Heizleitung SP1:":i16)
        n171 = Unbundle By Name(w187) -> ("Istwert"=→"Heizleitung SP2:":i16)
        n172 = Unbundle By Name(w188) -> ()  [unwired: 1 out]
        n173 = Index Array(array=w212) -> (element #1=→"Betriebsstunden Pumpe:":sgl, element #2=→"Betriebsstunden Anlage:":sgl)  [unwired: 2 in]
        n174 = call "FGV FT-IR Diagnosewerte.vi"("Aktionen"=FGV_FT-IR_Diagnose_Aktionen."Lesen") -> ("Druck"=→"Eingangsdruck FT-IR:":dbl, "Temperatur"=→"Temp. Messzelle:":dbl)  [unwired: 5 in, 4 out]
        n175 = Select(t=T11."Enabled", s=w209, f=T11."Disabled and Grayed Out" ("Deaktiviert")) -> (s? t:f=w208:T11)
        n176 = property on="Druck CalGas:" class="DigWert (strikt)"("DisabledEnum"=w208) -> (error out=w207:errorcluster)  [unwired: 2 in, 1 out]
        n177 = Index Array(array=w199) -> (element #1=→"H2O":sgl, element #2=→"O2":sgl, element #3=→"HC":sgl)  [unwired: 3 in]
        n178 = call "FGV Ventile manuell schalten Crio.vi"("Aktion"=Aktion_FGV_Ventile_manuell_schalten_Crio."lesen") -> ("Betrieb"=w178:u16)  [unwired: 11 in, 3 out]
        n179 = local write "Manueller Betrieb"(w178) -> ()
        n180 = call "Uebersicht Ausgabefelder einfaerben.vi"("Aktionen"=Aktionen_Ausgabefaelder_einfaerben."prüfen") -> ()  [unwired: 11 in]
        n181 = call <vilib>:"Clear Errors.vi"("error in (no error)"=w207) -> ()  [unwired: 5 in, 2 out]
      }
      event "20Y1", "20Y2", "20Y3", "20Y4", "20Y5", "20Y6", "20Y7", "20Y8", "21Y1", "21Y5", "21Y6", "22Y1", "22Y2", "23Y6", "23Y3", "23Y4": Value Change {
        n182 = event-data() -> ()  [unwired: 1 in, 1 out]
        n183 = call "FGV Ventile manuell schalten Crio.vi"("Aktion"=Aktion_FGV_Ventile_manuell_schalten_Crio."lesen") -> ("Betrieb"=w273:u16)  [unwired: 11 in, 3 out]
        n184 = case shown="1" w273 {
          frame 0, Default {
          }
          frame 1 {
            n185 = Build Array("20Y1", "20Y2", "20Y3", "20Y4", "20Y5", "20Y6", "20Y7", "20Y8", "21Y1", "21Y5", "21Y6", "22Y1", "22Y2", "23Y3", "23Y4", "23Y6") -> (w276:bool[])
            n186 = Boolean Array To Number(Boolean array=w276) -> (number=w275:u32)
            n187 = call "FGV Ventile manuell schalten Crio.vi"("Ventile schalten"=w275, "Aktion"=Aktion_FGV_Ventile_manuell_schalten_Crio."Ventile schalten") -> ()  [unwired: 10 in, 4 out]
          }
        }
      }
      event "CG-Test": Value Change {
        n188 = event-data() -> ()  [unwired: 1 in, 6 out]
        n189 = vi-ref "Erweiterte Konfig.lvlib:CG-Check Konfig.lvlib:CG-Test.vi"() -> (w294:refnum<vi>)
        n190 = call "VI Pop Up.vi"("VI Referenz"=w294) -> ()  [unwired: 10 in, 1 out]
      }
      event "N2 zu PNS": Value Change {
        n191 = event-data() -> ()  [unwired: 1 in, 1 out]
        n192 = call "FGV-Erweiterte Bedienung.vi"("Aktion"=FGV_Erweiterte_Bedienung_Aktion."Lesen") -> ("N2 zu PNS"=w296:bool)  [unwired: 9 in, 1 out]
        n193 = Not(x=w296) -> (.not. x?=w295:bool)
        n194 = call "FGV-Erweiterte Bedienung.vi"("Aktion"=FGV_Erweiterte_Bedienung_Aktion."N2 zu PNS", "N2 zu PNS"=w295) -> ()  [unwired: 8 in, 2 out]
      }
      event "VFS": Value Change {
        n195 = event-data() -> ()  [unwired: 1 in, 1 out]
        n196 = disable-structure shown="Amium_PNS_aktiv==FALSE, Standard" {
          disable-tunnel: [w300 w301] -> w299
          frame condition #0 {
            n197 = vi-ref "Amium PNS.lvlib:Anlagenuebersicht_amium2.vi"() -> (w300:refnum<vi>)
          }
          frame condition #1 (active) {
            n198 = vi-ref "PNS.lvlib:PNS Anlagenuebersicht.lvlib:VisBx Anzeige PNS.vi"() -> (w301:refnum<vi>)
          }
        }
        n199 = call "VI Pop Up.vi"("VI Referenz"=w299) -> ()  [unwired: 10 in, 1 out]
      }
      event "Manueller Betrieb": Value Change {
        n200 = event-data() -> ()  [unwired: 1 in, 1 out]
        n201 = case shown="1" "Manueller Betrieb" {
          frame 0, Default {
            n202 = call "FGV Ventile manuell schalten Crio.vi"("Aktion"=Aktion_FGV_Ventile_manuell_schalten_Crio."Testbetrieb inaktiv") -> ()  [unwired: 11 in, 4 out]
          }
          frame 1 {
            # "Schalter Initialisieren"
            # "HP"
            n203 = call "FGV-Funktionstasten.vi"("Aktion"=Funktionstasten-Aktion."Lesen") -> ("Samplepoint"=w307:u16, "ausgewählte Funktion"=w308:T39)  [unwired: 7 in, 6 out]
            n204 = call "Loopkennung.vi"("Aktion"=Aktionen_FGV_Loopkennung."lesen") -> ("LoopGeraetekennung"=w337:T40)  [unwired: 9 in, 1 out]
            n205 = call "FGV cRIO-Daten.vi"("Aktion"=enum16{"lesen", "schreiben"}."lesen") -> ("DO 0-31"=w331:T38)  [unwired: 9 in, 9 out]
            n206 = Unbundle By Name(w337) -> ("LP Kennung"=w336:u16)
            n207 = call "FGV-Funktionstasten.vi"("Samplepoint"=w307, "Herkunft"="Valve manuel switching", "Zustand"=w308, "Aktion"=Funktionstasten-Aktion."Zustand setzen") -> ("Fehler steht an"=w305:bool)  [unwired: 4 in, 7 out]
            n208 = Unbundle By Name(w331) -> ("O0: Druckluft Versorgung"=w330:bool, "O1: CG 1 (FB Eingang 1)"=w329:bool, "O2: CG 2 (Kühlung FT-IR EIN)"=w328:bool, "O3: CG 3 (FB Bypass)"=w327:bool, "O4: CG 4 (FB CalGas)"=w326:bool, "O5: CG 5 (FB spülen/UL)"=w325:bool, "O6: CG 6 (FB zum FT-IR)"=w324:bool, "O7: CG 7 (FB zum FID)"=w323:bool, "O8: CG 8 (FB Reserve)"=w322:bool, "O12: FB Stickstoff zu FT-IR"=w321:bool, "O13: Optikbox FT-IR spülen"=w320:bool, "O16: N2 Einblasung"=w319:bool, "O17: LSP LN2 Nachfüllung"=w318:bool, "O24: CalGas 1"=w317:bool, "O25: CalGas 2"=w316:bool, "O29: FTIR Standby Spülung"=w315:bool)
            n209 = call "FGV Grenzwerte PNS.vi"("Aktionen FGV Grenzwerte"=Aktionen_FGV_Grenzwerte."lesen") -> ("Anweisungscode"=w334:u16)  [unwired: 12 in, 2 out]
            n210 = Greater Than 0?(x=w336) -> (x > 0?=w335:bool)
            n211 = case shown="False" w335 {
              tunnel: w334 -> [w349 w369]
              tunnel: [w348 w368] -> w304
              tunnel: w305 -> [_ _]
              frame True {
                # "LP"
                n212 = case shown="17" w349 {
                  tunnel: [u32 0 ("Ventile schalten") u32 0 ("Ventile schalten") u32 0 ("Ventile schalten") u32 1025 ("Ventile schalten") u32 1040 ("Ventile schalten") u32 1030 ("Ventile schalten") u32 17 ("Ventile schalten") u32 2 ("Ventile schalten") u32 1056 ("Ventile schalten") u32 33 ("Ventile schalten") u32 1088 ("Ventile schalten") u32 65 ("Ventile schalten") u32 1152 ("Ventile schalten") u32 129 ("Ventile schalten") u32 1280 ("Ventile schalten") u32 257 ("Ventile schalten") u32 1536 ("Ventile schalten") u32 513 ("Ventile schalten")] -> w348
                  frame 0, Default {
                  }
                  frame 1 {
                  }
                  frame 2 {
                  }
                  frame 3 {
                  }
                  frame 4 {
                  }
                  frame 5 {
                  }
                  frame 6 {
                  }
                  frame 7 {
                  }
                  frame 8 {
                  }
                  frame 9 {
                  }
                  frame 10 {
                  }
                  frame 11 {
                  }
                  frame 12 {
                  }
                  frame 13 {
                  }
                  frame 14 {
                  }
                  frame 15 {
                  }
                  frame 16 {
                  }
                  frame 17 {
                  }
                }
              }
              frame False {
                # "HP"
                n213 = case shown="2" w369 {
                  tunnel: [u32 0 ("Ventile schalten") u32 0 ("Ventile schalten") u32 0 ("Ventile schalten") u32 4 ("Ventile schalten") u32 16 ("Ventile schalten") u32 6 ("Ventile schalten") u32 17 ("Ventile schalten") u32 2 ("Ventile schalten") u32 32 ("Ventile schalten") u32 33 ("Ventile schalten") u32 64 ("Ventile schalten") u32 65 ("Ventile schalten") u32 128 ("Ventile schalten") u32 129 ("Ventile schalten") u32 256 ("Ventile schalten") u32 257 ("Ventile schalten") u32 512 ("Ventile schalten") u32 513 ("Ventile schalten")] -> w368
                  frame 0, Default {
                  }
                  frame 1 {
                  }
                  frame 2 {
                  }
                  frame 3 {
                  }
                  frame 4 {
                  }
                  frame 5 {
                  }
                  frame 6 {
                  }
                  frame 7 {
                  }
                  frame 8 {
                  }
                  frame 9 {
                  }
                  frame 10 {
                  }
                  frame 11 {
                  }
                  frame 12 {
                  }
                  frame 13 {
                  }
                  frame 14 {
                  }
                  frame 15 {
                  }
                  frame 16 {
                  }
                  frame 17 {
                  }
                }
              }
            }
            n214 = Number To Boolean Array(number=w304) -> (Boolean array=w346:bool[])
            n215 = Index Array(array=w346) -> (element #1=w347:bool, element #2=w345:bool, element #3=w344:bool, element #5=w343:bool, element #6=w342:bool, element #7=w341:bool, element #8=w340:bool, element #12=w311:bool)  [unwired: 12 in, 4 out]
            n216 = local write "20Y1"(w330) -> ()
            n217 = local write "20Y2"(w329) -> ()
            n218 = local write "20Y3"(w328) -> ()
            n219 = local write "20Y4"(w327) -> ()
            n220 = local write "20Y5"(w326) -> ()
            n221 = local write "20Y6"(w325) -> ()
            n222 = local write "20Y7"(w324) -> ()
            n223 = local write "20Y8"(w323) -> ()
            n224 = local write "21Y1"(w322) -> ()
            n225 = local write "21Y5"(w321) -> ()
            n226 = local write "21Y6"(w320) -> ()
            n227 = local write "22Y1"(w319) -> ()
            n228 = local write "22Y2"(w318) -> ()
            n229 = local write "23Y3"(w317) -> ()
            n230 = local write "23Y4"(w316) -> ()
            n231 = local write "23Y6"(w315) -> ()
            n232 = call "FGV Ventile manuell steuern.vi"("Ventile schalten"=w304, "Aktion"=Aktion_FGV_Ventile_manuell_steuern."Ventile schalten") -> ()  [unwired: 12 in, 2 out]
            n233 = local write "12Y1"(w347) -> ()
            n234 = local write "11Y2"(w345) -> ()
            n235 = local write "11Y3"(w344) -> ()
            n236 = local write "11Y5"(w343) -> ()
            n237 = local write "11Y6"(w342) -> ()
            n238 = local write "Eingang 3"(w341) -> ()
            n239 = local write "Eingang 4"(w340) -> ()
            n240 = local write "11Y7"(w311) -> ()
            n241 = call "FGV Ventile manuell schalten Crio.vi"("Ventile schalten"=w304, "Aktion"=Aktion_FGV_Ventile_manuell_schalten_Crio."Testbetrieb aktiv") -> ()  [unwired: 10 in, 4 out]
            n242 = call "FGV Grenzwerte PNS.vi"("Anweisungscode"=u16 99, "Samplepoint"=w304, "Aktionen FGV Grenzwerte"=Aktionen_FGV_Grenzwerte."Anweisungscode vorgeben") -> ()  [unwired: 10 in, 3 out]
          }
        }
      }
      event "12Y1", "11Y2", "11Y3", "11Y6", "Eingang 3", "Eingang 4", "11Y7", "11Y5": Value Change {
        w388 = FALSE ("Element")
        n243 = event-data() -> ()  [unwired: 1 in, 1 out]
        n244 = Build Array("12Y1", "11Y2", "11Y3", w388, "11Y5", "11Y6", "Eingang 3", "Eingang 4", w388, w388, w388, "11Y7") -> (w399:bool[])
        n245 = Boolean Array To Number(Boolean array=w399) -> (number=w390:u32)
        n246 = call "FGV Ventile manuell steuern.vi"("Ventile schalten"=w390, "Aktion"=Aktion_FGV_Ventile_manuell_steuern."Ventile schalten") -> ()  [unwired: 12 in, 2 out]
      }
    }
  }
  n247 = disable-structure shown="Deaktiviert" {
    frame Disabled {
      n248 = flat-sequence {
        frame #0 {
          w400 = TRUE ("Sichtbar")
          n249 = property on="HL Ext.:" class="DigWert (strikt)"("Visible"=w400) -> ()  [unwired: 2 in, 2 out]
          n250 = property on="Druck CalGas:" class="DigWert (strikt)"("Visible"=w400) -> ()  [unwired: 2 in, 2 out]
        }
      }
    }
    frame Enabled {
    }
  }
